vi "3.1-Act UDP.vi"() -> ()   [LabVIEW 2010]
uses:
  4-High Neurons/4.1-Act Control Typedef.ctl
  4-High Neurons/4.1.0-Datatype Typedef.ctl
  4-High Neurons/4.1.1-Act Joystick.ctl
  4-High Neurons/4.1.2-Act Neuron TD.ctl
  3.0-Global.vi
panel:
  out "error out":errorcluster
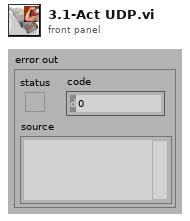
[diagram p1: front panel]
types:
  T1 = typedef "4.1-Act Control Typedef.ctl" = cluster{"4.1.0 Data":variant, "Type of Data":T2, "E-Stop":bool, "Restart":bool, "New IP":bool, "Begin":bool, "Time":i32, "Shutdown":bool}
  T2 = typedef "4.1.0-Datatype Typedef.ctl" = enum16{"4.1.0-Empty Data", "4.1.1-Joystick Data", "4.1.2-Behavioral Data"}
  T3 = typedef "4.1.1-Act Joystick.ctl" = cluster{"Trig":bool, "2":bool, "3":bool, "4":bool, "5":bool, "6":bool, "7":bool, "8":bool, "9":bool, "10":bool, "11":bool, "Pitch":i32, "Ang":bool[], "Wheel":dbl, "Roll":i32, "Yaw":i32, "Left":i32, "Right":i32}
  T4 = typedef "4.1.2-Act Neuron TD.ctl" = cluster{"Speed By Path":dbl[]}
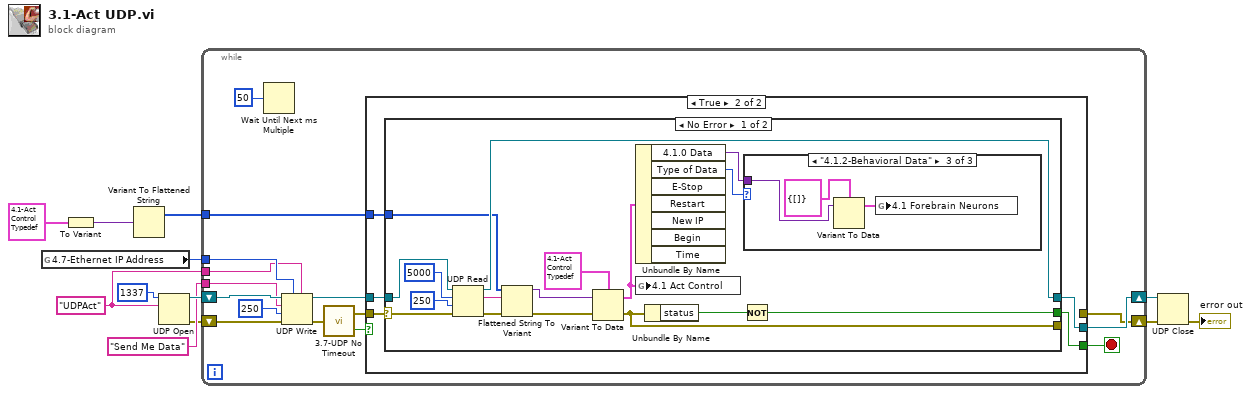
[diagram p0: block diagram]
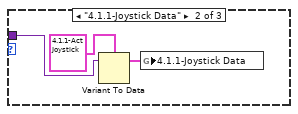
[diagram p4: hidden frame]
diagram:
  w1 = "UDPAct"
  n1 = global read "3.0-Global.vi" "4.7-Ethernet IP Address"() -> (w2:u32)
  n2 = To Variant(anything=T1 {"4.1.0 Data"=variant, "Type of Data"=enum."4.1.0-Empty Data", "E-Stop"=FALSE, "Restart"=FALSE, "New IP"=FALSE, "Begin"=FALSE, "Time"=0, "Shutdown"=FALSE} ("4.1 Act Control")) -> (Variant=w12:variant)
  n3 = Variant To Flattened String(Variant=w12) -> (1:w9:i16[])  [unwired: 1 out]
  n4 = UDP Open(10:w1, 11:u16 1337 ("port")) -> (port=w10:refnum<k16>, 0:w3:errorcluster)  [unwired: 3 in, 1 out]
  n5 = while {
    shift-right: [w25] -> w7
    shift-left: w10 -> [w26]
    tunnel: w9 -> [w24]
    shift-right: [w23] -> w6
    shift-left: w3 -> [w21]
    tunnel: "Send Me Data" -> [w22]
    tunnel: w2 -> [w14]
    tunnel: w1 -> [w13]
    stop <- w27 stop-if-true
    n6 = Wait Until Next ms Multiple(millisecond multiple=u32 50) -> ()  [unwired: 1 out]
    n7 = UDP Write(address=w14, port or service name=w13, connection ID=w26, data in=w22, 8:w21, 9:250 ("timeout ms (25000)")) -> (error out=w19:errorcluster, 3:w17:refnum<k16>)
    n8 = call "3.7-UDP No Timeout.vi"("error in (no error)"=w19) -> ("No Timeout"=w16:bool, "error out"=w15:errorcluster)
    n9 = case shown="True" w16 {
      tunnel: w15 -> [w29 w30]
      tunnel: w17 -> [w28 w34]
      tunnel: [w28 w33] -> w25
      tunnel: [w29 _] -> w23
      tunnel: w24 -> [_ w32]
      tunnel: [_ w31] -> w27
      frame False {
      }
      frame True {
        n10 = case shown="No Error" w30 {
          selector: w30 -> [w51 w58]
          tunnel: w34 -> [w50 w59]
          tunnel: [w48 w59] -> w33
          tunnel: [w41 w58] -> _
          tunnel: w32 -> [w45 _]
          tunnel: [w39 _] -> w31
          frame No Error {
            n11 = UDP Read(connection ID=w50, max size (548)=5000, timeout ms (25000)=250, 8:w51) -> (data out=w46:string, error out=w42:errorcluster, 3:w48:refnum<k16>)  [unwired: 2 out]
            n12 = Flattened String To Variant(4:w42, 6:w46, 7:w45) -> (0:w43:errorcluster, 3:w44:variant)
            n13 = Variant To Data(error in=w43, Variant=w44, type=T1 {"4.1.0 Data"=variant, "Type of Data"=enum."4.1.1-Joystick Data", "E-Stop"=FALSE, "Restart"=FALSE, "New IP"=FALSE, "Begin"=FALSE, "Time"=0, "Shutdown"=FALSE} ("4.1 Act Control")) -> (error out=w41:errorcluster, data=w35:T1)
            n14 = Unbundle By Name(w35) -> ("4.1.0 Data"=w37:variant, "Type of Data"=w38:T2)  [unwired: 5 out]
            n15 = global write "3.0-Global.vi" "4.1 Act Control"(w35) -> ()
            n16 = Unbundle By Name(w41) -> ("status"=w40:bool)
            n17 = Not(x=w40) -> (.not. x?=w39:bool)
            n18 = case shown="\"4.1.2-Behavioral Data\"" w38 {
              tunnel: w37 -> [_ w54 w57]
              frame "4.1.0-Empty Data", Default {
              }
              frame "4.1.1-Joystick Data" {
                n19 = Variant To Data(Variant=w54, type=T3 {"Trig"=FALSE, "2"=FALSE, "3"=FALSE, "4"=FALSE, "5"=FALSE, "6"=FALSE, "7"=FALSE, "8"=FALSE, "9"=FALSE, "10"=FALSE, "11"=FALSE, "Pitch"=0, "Ang"=[], "Wheel"=0.0, "Roll"=0, "Yaw"=0, "Left"=0, "Right"=0} ("Saitek Controler")) -> (data=w52:T3)  [unwired: 1 in, 1 out]
                n20 = global write "3.0-Global.vi" "4.1.1-Joystick Data"(w52) -> ()
              }
              frame "4.1.2-Behavioral Data" {
                n21 = Variant To Data(Variant=w57, type=T4 {"Speed By Path"=[]} ("Forebrain Act Neurons")) -> (data=w55:T4)  [unwired: 1 in, 1 out]
                n22 = global write "3.0-Global.vi" "4.1 Forebrain Neurons"(w55) -> ()
              }
            }
          }
          frame Error {
          }
        }
      }
    }
  }
  n23 = UDP Close(connection ID=w7, 8:w6) -> (error out=→"error out":errorcluster)  [unwired: 1 out]
